vi "Lab Panel V6.00.vi"() -> ()   [LabVIEW 2017] (continued)
                            n1789 = local write "mail control"("END") -> ()
                            n1790 = Bundle(cluster=w3343) -> (w3344:T4)  [unwired: 3 in]
                            n1791 = local write "RUN LAB05-2"(w3341) -> ()
                            n1792 = local write "O/I  LAB05-2"(w3341) -> ()
                            n1793 = local write "run lab05-2"(w3341) -> ()
                            n1794 = local write "DISP LAB05-2"(w3344) -> ()
                          }
                          frame #1 {
                            n1795 = TDMS Close(11:w3345) -> (0:w3346:errorcluster)  [unwired: 1 in, 1 out]
                            n1796 = local write "data file error"(w3346) -> ()
                          }
                          frame #2 {
                            n1797 = stacked-sequence {
                              tunnel: "LAB05-2" -> [w3354 w3360]
                              tunnel: w3351 -> [_ w3359]
                              tunnel: w3350 -> [_ w3358]
                              tunnel: w3349 -> [_ w3357]
                              tunnel: w3348 -> [_ w3356]
                              tunnel: w3347 -> [_ w3355]
                              frame #0 {
                                n1798 = call "sub vi - defrag tdms v1.vi"("panel id"=w3354) -> ("error out"=w3353:errorcluster)  [unwired: 10 in]
                                n1799 = local write "data file error"(w3353) -> ()
                              }
                              frame #1 {
                                n1800 = Bundle("STATUS"=w3359, "OUT SERVER ADDRESS"=w3358, "FROM ACCOUNT"=w3357, "Mail Test File To:"=w3356, "Mail Test Fail"=w3355) -> (w3362:T29)  [unwired: 1 in]
                                n1801 = call "Save data file (pass-fail) v5.vi"("Input Cluster"=w3362, "panel id"=w3360) -> ("network file save error"=w3361:errorcluster)  [unwired: 8 in, 1 out]
                                n1802 = local write "data file error"(w3361) -> ()
                              }
                            }
                          }
                        }
                      }
                    }
                  }
                }
              }
            }
            n1803 = global write "Global display 2.vi" "Mail test file to:"(w2869) -> ()
            n1804 = local read "Network Directory"() -> (w2875:path)
            n1805 = global write "Global 1.vi" "Network Drive"(w2875) -> ()
          }
          frame #8 {
            # "disable functions"
            n1806 = stacked-sequence {
              tunnel: w3372 -> [w3386 _ w3443]
              tunnel: w3371 -> [w3381 _ w3442]
              tunnel: w3370 -> [w3380 _ w3441]
              tunnel: w3369 -> [w3378 _ w3440]
              tunnel: w3368 -> [w3379 _ w3439]
              tunnel: w3367 -> [_ w3403 w3438]
              tunnel: w3366 -> [_ w3404 w3437]
              tunnel: w3365 -> [_ w3405 w3436]
              tunnel: w3364 -> [_ w3406 w3435]
              tunnel: w3363 -> [_ w3407 w3434]
              frame #0 {
                n1807 = Select(t=2, s=w3378, f=0) -> (s? t:f=w3374:i32)
                n1808 = Select(t=2, s=w3380, f=0) -> (s? t:f=w3375:i32)
                n1809 = Select(t=2, s=w3379, f=0) -> (s? t:f=w3373:i32)
                n1810 = Select(t=2, s=w3386, f=0) -> (s? t:f=w3377:i32)
                n1811 = Select(t=2, s=w3381, f=0) -> (s? t:f=w3376:i32)
                n1812 = property on="SELECT LAB02-2" class="RadioBtnsControl (strict)"("DisabledEnum"=w3374) -> ()  [unwired: 2 in, 2 out]
                n1813 = property on="SELECT LAB02-1" class="RadioBtnsControl (strict)"("DisabledEnum"=w3375) -> ()  [unwired: 2 in, 2 out]
                n1814 = property on="SELECT LAB03-1" class="RadioBtnsControl (strict)"("DisabledEnum"=w3373) -> ()  [unwired: 2 in, 2 out]
                n1815 = property on="SELECT LAB01-1" class="RadioBtnsControl (strict)"("DisabledEnum"=w3377) -> ()  [unwired: 2 in, 2 out]
                n1816 = property on="SELECT LAB01-2" class="RadioBtnsControl (strict)"("DisabledEnum"=w3376) -> ()  [unwired: 2 in, 2 out]
                n1817 = Not(x=w3386) -> (.not. x?=w3387:bool)
                n1818 = property on="RESULT LAB01-1" class="Bool (strict)"("Visible"=w3387) -> ()  [unwired: 2 in, 2 out]
                n1819 = Not(x=w3381) -> (.not. x?=w3385:bool)
                n1820 = Not(x=w3380) -> (.not. x?=w3384:bool)
                n1821 = Not(x=w3378) -> (.not. x?=w3383:bool)
                n1822 = property on="RESULT LAB01-2" class="Bool (strict)"("Visible"=w3385) -> ()  [unwired: 2 in, 2 out]
                n1823 = Not(x=w3379) -> (.not. x?=w3382:bool)
                n1824 = property on="RESULT LAB02-1" class="Bool (strict)"("Visible"=w3384) -> ()  [unwired: 2 in, 2 out]
                n1825 = property on="RESULT LAB02-2" class="Bool (strict)"("Visible"=w3383) -> ()  [unwired: 2 in, 2 out]
                n1826 = property on="RESULT LAB03-1" class="Bool (strict)"("Visible"=w3382) -> ()  [unwired: 2 in, 2 out]
                n1827 = property on="SET LAB01-1" class="Clust (strict)"("DisabledEnum"=w3377) -> ()  [unwired: 2 in, 2 out]
                n1828 = property on="SET LAB01-2" class="Clust (strict)"("DisabledEnum"=w3376) -> ()  [unwired: 2 in, 2 out]
                n1829 = property on="SET LAB02-1" class="Clust (strict)"("DisabledEnum"=w3375) -> ()  [unwired: 2 in, 2 out]
                n1830 = property on="SET LAB02-2" class="Clust (strict)"("DisabledEnum"=w3374) -> ()  [unwired: 2 in, 2 out]
                n1831 = property on="SET LAB03-1" class="Clust (strict)"("DisabledEnum"=w3373) -> ()  [unwired: 2 in, 2 out]
                n1832 = property on="O/I  LAB01-1" class="Bool (strict)"("DisabledEnum"=w3377) -> ()  [unwired: 2 in, 2 out]
                n1833 = property on="O/I  LAB01-2" class="Bool (strict)"("DisabledEnum"=w3376) -> ()  [unwired: 2 in, 2 out]
                n1834 = property on="O/I  LAB02-1" class="Bool (strict)"("DisabledEnum"=w3375) -> ()  [unwired: 2 in, 2 out]
                n1835 = property on="O/I  LAB02-2" class="Bool (strict)"("DisabledEnum"=w3374) -> ()  [unwired: 2 in, 2 out]
                n1836 = property on="O/I  LAB03-1" class="Bool (strict)"("DisabledEnum"=w3373) -> ()  [unwired: 2 in, 2 out]
              }
              frame #1 {
                n1837 = Select(t=2, s=w3407, f=0) -> (s? t:f=w3398:i32)
                n1838 = Select(t=2, s=w3406, f=0) -> (s? t:f=w3399:i32)
                n1839 = Select(t=2, s=w3403, f=0) -> (s? t:f=w3402:i32)
                n1840 = Select(t=2, s=w3404, f=0) -> (s? t:f=w3401:i32)
                n1841 = Select(t=2, s=w3405, f=0) -> (s? t:f=w3400:i32)
                n1842 = property on="SELECT LAB05-2" class="RadioBtnsControl (strict)"("DisabledEnum"=w3398) -> ()  [unwired: 2 in, 2 out]
                n1843 = property on="SELECT LAB05-1" class="RadioBtnsControl (strict)"("DisabledEnum"=w3399) -> ()  [unwired: 2 in, 2 out]
                n1844 = property on="SELECT LAB03-2" class="RadioBtnsControl (strict)"("DisabledEnum"=w3402) -> ()  [unwired: 2 in, 2 out]
                n1845 = property on="SELECT LAB04-1" class="RadioBtnsControl (strict)"("DisabledEnum"=w3401) -> ()  [unwired: 2 in, 2 out]
                n1846 = property on="SELECT LAB04-2" class="RadioBtnsControl (strict)"("DisabledEnum"=w3400) -> ()  [unwired: 2 in, 2 out]
                n1847 = property on="SET LAB05-2" class="Clust (strict)"("DisabledEnum"=w3398) -> ()  [unwired: 2 in, 2 out]
                n1848 = property on="SET LAB05-1" class="Clust (strict)"("DisabledEnum"=w3399) -> ()  [unwired: 2 in, 2 out]
                n1849 = property on="SET LAB03-2" class="Clust (strict)"("DisabledEnum"=w3402) -> ()  [unwired: 2 in, 2 out]
                n1850 = property on="SET LAB04-1" class="Clust (strict)"("DisabledEnum"=w3401) -> ()  [unwired: 2 in, 2 out]
                n1851 = property on="SET LAB04-2" class="Clust (strict)"("DisabledEnum"=w3400) -> ()  [unwired: 2 in, 2 out]
                n1852 = property on="O/I  LAB05-2" class="Bool (strict)"("DisabledEnum"=w3398) -> ()  [unwired: 2 in, 2 out]
                n1853 = property on="O/I  LAB05-1" class="Bool (strict)"("DisabledEnum"=w3399) -> ()  [unwired: 2 in, 2 out]
                n1854 = property on="O/I  LAB04-1" class="Bool (strict)"("DisabledEnum"=w3401) -> ()  [unwired: 2 in, 2 out]
                n1855 = property on="O/I  LAB04-2" class="Bool (strict)"("DisabledEnum"=w3400) -> ()  [unwired: 2 in, 2 out]
                n1856 = property on="O/I  LAB03-2" class="Bool (strict)"("DisabledEnum"=w3402) -> ()  [unwired: 2 in, 2 out]
                n1857 = Not(x=w3407) -> (.not. x?=w3408:bool)
                n1858 = Not(x=w3406) -> (.not. x?=w3409:bool)
                n1859 = Not(x=w3405) -> (.not. x?=w3410:bool)
                n1860 = property on="RESULT LAB05-2" class="Bool (strict)"("Visible"=w3408) -> ()  [unwired: 2 in, 2 out]
                n1861 = property on="RESULT LAB05-1" class="Bool (strict)"("Visible"=w3409) -> ()  [unwired: 2 in, 2 out]
                n1862 = Not(x=w3404) -> (.not. x?=w3411:bool)
                n1863 = property on="RESULT LAB04-2" class="Bool (strict)"("Visible"=w3410) -> ()  [unwired: 2 in, 2 out]
                n1864 = Not(x=w3403) -> (.not. x?=w3412:bool)
                n1865 = property on="RESULT LAB04-1" class="Bool (strict)"("Visible"=w3411) -> ()  [unwired: 2 in, 2 out]
                n1866 = property on="RESULT LAB03-2" class="Bool (strict)"("Visible"=w3412) -> ()  [unwired: 2 in, 2 out]
              }
              frame #2 {
                # "disable calibrate if any test running"
                n1867 = Or(x=w3435, y=w3434) -> (x .or. y?=w3428:bool)
                n1868 = Or(x=w3437, y=w3436) -> (x .or. y?=w3430:bool)
                n1869 = Or(x=w3441, y=w3440) -> (x .or. y?=w3432:bool)
                n1870 = Or(x=w3439, y=w3438) -> (x .or. y?=w3431:bool)
                n1871 = Or(x=w3443, y=w3442) -> (x .or. y?=w3433:bool)
                n1872 = Or(x=w3431, y=w3430) -> (x .or. y?=w3429:bool)
                n1873 = Or(x=w3433, y=w3432) -> (x .or. y?=w3427:bool)
                n1874 = Or(x=w3429, y=w3428) -> (x .or. y?=w3426:bool)
                n1875 = Or(x=w3427, y=w3426) -> (x .or. y?=w3423:bool)
                "Any Test Running" <- w3423
                n1876 = case shown="False" w3423 {
                  tunnel: [0 2] -> w3425
                  frame False {
                  }
                  frame True {
                  }
                }
                n1877 = property on="JIG TEST" class="Clust (strict)"("DisabledEnum"=w3425) -> ()  [unwired: 2 in, 2 out]
                n1878 = property on="Network Directory" class="Path"("DisabledEnum"=w3425) -> ()  [unwired: 2 in, 2 out]
                n1879 = property on="MAIL SETTINGS" class="Clust (strict)"("DisabledEnum"=w3425) -> ()  [unwired: 2 in, 2 out]
                n1880 = property on="SET (cal)" class="Bool (strict)"("DisabledEnum"=w3425) -> ()  [unwired: 2 in, 2 out]
                n1881 = property on="ADMIN" class="Bool (strict)"("DisabledEnum"=0) -> ()  [unwired: 2 in, 2 out]
              }
            }
          }
          frame #9 {
            # "Note : JIG LAB0X-N   are written to digital I/O in frame 11"
            # "Drive jigs"
            n1882 = stacked-sequence {
              frame #0 {
                # "jig on"
                n1883 = local read "jig cycle"() -> (w3451:dbl)
                n1884 = property on="JIG TEST" class="Clust (strict)"() -> ("DisabledEnum"=w3448:T17)  [unwired: 2 in, 2 out]
                n1885 = Equal?(x=w3448, y=2) -> (x = y?=w3447:bool)
                n1886 = Equal?(x=w3451, y=0) -> (x = y?=w3449:bool)
                n1887 = And(x=w3449, y=w3447) -> (x .and. y?=w3446:bool)
                n1888 = case shown="True" w3446 {
                  frame False {
                  }
                  frame True {
                    n1889 = local read "run lab01-2"() -> (w3461:bool)
                    n1890 = local read "run lab01-1"() -> (w3462:bool)
                    n1891 = local read "run lab02-1"() -> (w3460:bool)
                    n1892 = local read "run lab02-2"() -> (w3459:bool)
                    n1893 = local read "run lab03-1"() -> (w3458:bool)
                    n1894 = local read "run lab03-2"() -> (w3457:bool)
                    n1895 = local read "run lab04-1"() -> (w3456:bool)
                    n1896 = local read "run lab04-2"() -> (w3455:bool)
                    n1897 = local read "run lab05-1"() -> (w3454:bool)
                    n1898 = local read "run lab05-2"() -> (w3453:bool)
                    n1899 = local write "JIG LAB01-2"(w3461) -> ()
                    n1900 = local write "JIG LAB03-2"(w3457) -> ()
                    n1901 = local write "JIG LAB01-1"(w3462) -> ()
                    n1902 = local write "JIG LAB02-1"(w3460) -> ()
                    n1903 = local write "JIG LAB02-2"(w3459) -> ()
                    n1904 = local write "JIG LAB03-1"(w3458) -> ()
                    n1905 = local write "JIG LAB04-1"(w3456) -> ()
                    n1906 = local write "JIG LAB04-2"(w3455) -> ()
                    n1907 = local write "JIG LAB05-1"(w3454) -> ()
                    n1908 = local write "JIG LAB05-2"(w3453) -> ()
                  }
                }
              }
              frame #1 {
                # "jig off"
                n1909 = local read "jig cycle"() -> (w3469:dbl)
                n1910 = local read "on loops"() -> (w3468:dbl)
                n1911 = property on="JIG TEST" class="Clust (strict)"() -> ("DisabledEnum"=w3467:T17)  [unwired: 2 in, 2 out]
                n1912 = Equal?(x=w3467, y=2) -> (x = y?=w3465:bool)
                n1913 = Equal?(x=w3469, y=w3468) -> (x = y?=w3464:bool)
                n1914 = And(x=w3464, y=w3465) -> (x .and. y?=w3463:bool)
                n1915 = case shown="True" w3463 {
                  frame False {
                  }
                  frame True {
                    w3520 = FALSE
                    w3521 = TRUE
                    w3519 = 2
                    n1916 = local read "SELECT LAB05-2"() -> (w3510:T3)
                    n1917 = local read "SELECT LAB04-2"() -> (w3512:T3)
                    n1918 = local read "SELECT LAB04-1"() -> (w3513:T3)
                    n1919 = local read "SELECT LAB05-1"() -> (w3511:T3)
                    n1920 = local read "SELECT LAB03-2"() -> (w3514:T3)
                    n1921 = local read "SELECT LAB02-1"() -> (w3517:T3)
                    n1922 = local read "SELECT LAB03-1"() -> (w3515:T3)
                    n1923 = local read "SELECT LAB02-2"() -> (w3516:T3)
                    n1924 = local read "SELECT LAB01-2"() -> (w3518:T3)
                    n1925 = local read "run lab05-1"() -> (w3480:bool)
                    n1926 = local read "run lab05-2"() -> (w3479:bool)
                    n1927 = local read "run lab04-2"() -> (w3481:bool)
                    n1928 = local read "SELECT LAB01-1"() -> (w3522:T3)
                    n1929 = local read "run lab04-1"() -> (w3482:bool)
                    n1930 = local read "run lab01-1"() -> (w3498:bool)
                    n1931 = local read "run lab01-2"() -> (w3487:bool)
                    n1932 = local read "run lab03-2"() -> (w3483:bool)
                    n1933 = local read "run lab03-1"() -> (w3484:bool)
                    n1934 = local read "run lab02-1"() -> (w3486:bool)
                    n1935 = local read "run lab02-2"() -> (w3485:bool)
                    n1936 = Equal?(x=w3519, y=w3515) -> (x = y?=w3493:bool)
                    n1937 = Equal?(x=w3519, y=w3514) -> (x = y?=w3492:bool)
                    n1938 = Equal?(x=w3519, y=w3513) -> (x = y?=w3491:bool)
                    n1939 = Equal?(x=w3519, y=w3512) -> (x = y?=w3490:bool)
                    n1940 = Equal?(x=w3519, y=w3511) -> (x = y?=w3489:bool)
                    n1941 = Equal?(x=w3519, y=w3510) -> (x = y?=w3488:bool)
                    n1942 = Equal?(x=w3519, y=w3522) -> (x = y?=w3499:bool)
                    n1943 = Equal?(x=w3519, y=w3517) -> (x = y?=w3495:bool)
                    n1944 = Equal?(x=w3519, y=w3516) -> (x = y?=w3494:bool)
                    n1945 = Equal?(x=w3519, y=w3518) -> (x = y?=w3496:bool)
                    n1946 = And(x=w3490, y=w3481) -> (x .and. y?=w3472:bool)
                    n1947 = And(x=w3493, y=w3484) -> (x .and. y?=w3475:bool)
                    n1948 = And(x=w3491, y=w3482) -> (x .and. y?=w3473:bool)
                    n1949 = And(x=w3488, y=w3479) -> (x .and. y?=w3470:bool)
                    n1950 = And(x=w3494, y=w3485) -> (x .and. y?=w3476:bool)
                    n1951 = And(x=w3492, y=w3483) -> (x .and. y?=w3474:bool)
                    n1952 = And(x=w3489, y=w3480) -> (x .and. y?=w3471:bool)
                    n1953 = And(x=w3496, y=w3487) -> (x .and. y?=w3478:bool)
                    n1954 = And(x=w3499, y=w3498) -> (x .and. y?=w3497:bool)
                    n1955 = And(x=w3495, y=w3486) -> (x .and. y?=w3477:bool)
                    n1956 = Select(t=w3521, s=w3497, f=w3520) -> (s? t:f=w3500:bool)
                    n1957 = Select(t=w3521, s=w3478, f=w3520) -> (s? t:f=w3501:bool)
                    n1958 = Select(t=w3521, s=w3477, f=w3520) -> (s? t:f=w3502:bool)
                    n1959 = Select(t=w3521, s=w3476, f=w3520) -> (s? t:f=w3503:bool)
                    n1960 = Select(t=w3521, s=w3475, f=w3520) -> (s? t:f=w3504:bool)
                    n1961 = Select(t=w3521, s=w3474, f=w3520) -> (s? t:f=w3505:bool)
                    n1962 = Select(t=w3521, s=w3473, f=w3520) -> (s? t:f=w3506:bool)
                    n1963 = Select(t=w3521, s=w3472, f=w3520) -> (s? t:f=w3507:bool)
                    n1964 = Select(t=w3521, s=w3471, f=w3520) -> (s? t:f=w3508:bool)
                    n1965 = Select(t=w3521, s=w3470, f=w3520) -> (s? t:f=w3509:bool)
                    n1966 = local write "JIG LAB03-2"(w3505) -> ()
                    n1967 = local write "JIG LAB02-1"(w3502) -> ()
                    n1968 = local write "JIG LAB02-2"(w3503) -> ()
                    n1969 = local write "JIG LAB01-2"(w3501) -> ()
                    n1970 = local write "JIG LAB03-1"(w3504) -> ()
                    n1971 = local write "JIG LAB01-1"(w3500) -> ()
                    n1972 = local write "JIG LAB05-2"(w3509) -> ()
                    n1973 = local write "JIG LAB04-1"(w3506) -> ()
                    n1974 = local write "JIG LAB05-1"(w3508) -> ()
                    n1975 = local write "JIG LAB04-2"(w3507) -> ()
                  }
                }
              }
            }
          }
          frame #10 {
            # "Note : JIG LAB0X-N   are written to digital I/O in frame 11"
            # "enable  jig test output if no test busy"
            n1976 = property on="JIG TEST" class="Clust (strict)"() -> ("DisabledEnum"=w3525:T17)  [unwired: 2 in, 2 out]
            n1977 = Equal?(x=w3525, y=0) -> (x = y?=w3523:bool)
            n1978 = case shown="True" w3523 {
              frame False {
              }
              frame True {
                n1979 = local read "JIG TEST"() -> (w3536:T11)
                n1980 = Unbundle(w3536) -> ("LAB01-1"=w3535:bool, "LAB01-2"=w3534:bool, "LAB02-1"=w3533:bool, "LAB02-2"=w3532:bool, "LAB03-1"=w3531:bool, "LAB03-2"=w3530:bool, "LAB04-1"=w3529:bool, "LAB04-2"=w3528:bool, "LAB05-1"=w3527:bool, "LAB05-2"=w3526:bool)
                n1981 = local write "JIG LAB05-1"(w3527) -> ()
                n1982 = local write "JIG LAB05-2"(w3526) -> ()
                n1983 = local write "JIG LAB04-1"(w3529) -> ()
                n1984 = local write "JIG LAB04-2"(w3528) -> ()
                n1985 = local write "JIG LAB03-2"(w3530) -> ()
                n1986 = local write "JIG LAB01-1"(w3535) -> ()
                n1987 = local write "JIG LAB02-1"(w3533) -> ()
                n1988 = local write "JIG LAB03-1"(w3531) -> ()
                n1989 = local write "JIG LAB01-2"(w3534) -> ()
                n1990 = local write "JIG LAB02-2"(w3532) -> ()
              }
            }
          }
          frame #11 {
            w3537 = FALSE
            # "Drive digital output and reset USB and temperature network if required."
            n1991 = global read "Global display 3.vi" "cycle O/F"() -> (w3546:bool)
            n1992 = case shown="False" w3546 {
              tunnel: [w3678 FALSE] -> w3545
              frame False {
                n1993 = local read "Analog error"() -> (w3680:bool)
                n1994 = local read "Reset Measuring"() -> (w3679:bool)
                n1995 = Or(x=w3679, y=w3680) -> (x .or. y?=w3678:bool)
              }
              frame True {
              }
            }
            n1996 = local read "O/I  LAB01-1"() -> (w3565:bool)
            n1997 = local read "JIG LAB01-1"() -> (w3564:bool)
            n1998 = local read "O/I  LAB01-2"() -> (w3563:bool)
            n1999 = local read "JIG LAB01-2"() -> (w3562:bool)
            n2000 = local read "O/I  LAB02-1"() -> (w3561:bool)
            n2001 = local read "JIG LAB02-1"() -> (w3560:bool)
            n2002 = local read "O/I  LAB02-2"() -> (w3559:bool)
            n2003 = local read "JIG LAB02-2"() -> (w3558:bool)
            n2004 = local read "O/I  LAB03-1"() -> (w3557:bool)
            n2005 = local read "JIG LAB03-1"() -> (w3556:bool)
            n2006 = local read "O/I  LAB03-2"() -> (w3555:bool)
            n2007 = local read "JIG LAB03-2"() -> (w3554:bool)
            n2008 = local read "O/I  LAB04-1"() -> (w3553:bool)
            n2009 = local read "JIG LAB04-1"() -> (w3552:bool)
            n2010 = local read "O/I  LAB04-2"() -> (w3543:bool)
            n2011 = local read "JIG LAB04-2"() -> (w3542:bool)
            n2012 = local read "O/I  LAB05-1"() -> (w3541:bool)
            n2013 = local read "JIG LAB05-1"() -> (w3540:bool)
            n2014 = local read "O/I  LAB05-2"() -> (w3539:bool)
            n2015 = local read "JIG LAB05-2"() -> (w3538:bool)
            n2016 = Build Array(w3558, w3557, w3556, w3555, w3554, w3553, w3552) -> (w3550:bool[])
            "USB OUT 1" <- w3550
            n2017 = Build Array(w3565, w3564, w3563, w3562, w3561, w3560, w3559) -> (w3551:bool[])
            "USB OUT 0" <- w3551
            n2018 = Build Array(w3543, w3542, w3541, w3540, w3539, w3538, w3537, w3537) -> (w3549:bool[])
            "USB OUT 2" <- w3549
            n2019 = Not(x=w3546) -> (.not. x?=w3547:bool)
            n2020 = local read "Simulate"() -> (w3548:bool)
            n2021 = And(x=w3547, y=w3545) -> (x .and. y?=w3544:bool)
            n2022 = stacked-sequence {
              tunnel: w3551 -> [w3569 w3575]
              tunnel: w3550 -> [w3568 w3574]
              tunnel: w3549 -> [w3567 w3573]
              tunnel: w3548 -> [w3566 w3576]
              tunnel: w3544 -> [_ w3577]
              frame #0 {
                # "drive outputs for normal use"
                n2023 = case shown="False" w3566 {
                  tunnel: w3569 -> [w3572 _]
                  tunnel: w3568 -> [w3571 _]
                  tunnel: w3567 -> [w3570 _]
                  frame False {
                    n2024 = call "sub vi - Drive Relays All v6.vi"("Array #2"=w3570, "Array #1"=w3571, "Array #0"=w3572) -> ()  [unwired: 8 in, 1 out]
                  }
                  frame True {
                  }
                }
              }
              frame #1 {
                # "USB  reset routine"
                n2025 = case shown="True" w3577 {
                  tunnel: w3576 -> [_ w3581]
                  tunnel: w3575 -> [_ w3580]
                  tunnel: w3574 -> [_ w3579]
                  tunnel: w3573 -> [_ w3578]
                  frame False {
                  }
                  frame True {
                    n2026 = stacked-sequence {
                      seq-local: [w3583 _ _ _ _] -> [_ w3589 _ _ _]
                      tunnel: w3581 -> [_ w3593 _ _ _]
                      tunnel: w3580 -> [_ w3592 _ _ _]
                      tunnel: w3579 -> [_ w3591 _ _ _]
                      tunnel: w3578 -> [_ w3590 _ _ _]
                      frame #0 {
                        n2027 = case shown="False" "Auto Reset" {
                          tunnel: [w3586 FALSE] -> w3584
                          frame False {
                            n2028 = Two Button Dialog(message="System reset") -> (T button?=w3586:bool)  [unwired: 2 in]
                          }
                          frame True {
                          }
                        }
                        n2029 = disable-structure shown="Disabled" {
                          frame Disabled {
                            n2030 = local write "Tab Control 2"(5) -> ()
                          }
                          frame Enabled {
                          }
                        }
                        n2031 = Or(x="Auto Reset", y=w3584) -> (x .or. y?=w3583:bool)
                      }
                      frame #1 {
                        n2032 = case shown="True" w3589 {
                          tunnel: w3593 -> [_ w3599]
                          tunnel: w3592 -> [_ w3598]
                          tunnel: w3591 -> [_ w3597]
                          tunnel: w3590 -> [_ w3596]
                          frame False {
                          }
                          frame True {
                            n2033 = stacked-sequence {
                              tunnel: w3599 -> [_ w3617 _]
                              tunnel: bool[] [] -> [w3602 w3616 w3635]
                              tunnel: w3598 -> [_ _ w3634]
                              tunnel: w3597 -> [w3601 _ w3633]
                              tunnel: w3596 -> [w3600 _ w3632]
                              tunnel: 5000 -> [w3603 _ w3631]
                              frame #0 {
                                # "switch off test stations for system reset"
                                n2034 = stacked-sequence {
                                tunnel: w3603 -> [w3607 w3611 w3613]
                                tunnel: w3602 -> [w3606 w3610 w3614]
                                tunnel: w3601 -> [w3605 _ _]
                                tunnel: w3600 -> [w3604 w3609 _]
                                frame #0 {
                                # "drive 1st 7 inputs"
                                n2035 = call "sub vi - Drive Relays All v6.vi"("Array #2"=w3604, "Array #1"=w3605, "Array #0"=w3606) -> ()  [unwired: 8 in, 1 out]
                                n2036 = call "Message Display V1.vi"("Message"="Delay off LAB 01-1 to 02-1", "Delay mS"=w3607) -> ()  [unwired: 10 in]
                                }
                                frame #1 {
                                # "drive 2nd 7 inputs"
                                n2037 = call "sub vi - Drive Relays All v6.vi"("Array #2"=w3609, "Array #1"=w3610, "Array #0"=w3610) -> ()  [unwired: 8 in, 1 out]
                                n2038 = call "Message Display V1.vi"("Message"="Delay off LAB 02-2 to 04-1", "Delay mS"=w3611) -> ()  [unwired: 10 in]
                                }
                                frame #2 {
                                # "drive 3rd 7 inputs"
                                n2039 = call "sub vi - Drive Relays All v6.vi"("Array #2"=w3614, "Array #1"=w3614, "Array #0"=w3614) -> ()  [unwired: 8 in, 1 out]
                                n2040 = call "Message Display V1.vi"("Message"="Delay off LAB 04-2 to 05-2", "Delay mS"=w3613) -> ()  [unwired: 10 in]
                                }
                                }
                              }
                              frame #1 {
                                # "reset all usb modules"
                                n2041 = stacked-sequence {
                                tunnel: w3617 -> [_ w3622]
                                tunnel: w3616 -> [w3620 _]
                                frame #0 {
                                n2042 = local write "AI Task"(FALSE) -> ()
                                n2043 = call "sub vi - Drive Relays All v6.vi"("Array #2"=bool[] [FALSE, FALSE, FALSE, FALSE, FALSE, FALSE, TRUE, FALSE], "Array #1"=w3620, "Array #0"=w3620) -> ()  [unwired: 8 in, 1 out]
                                }
                                frame #1 {
                                n2044 = call "Reset Meas v 5.vi"("simulate"=w3622) -> ("Reset Error"=w3621:bool)  [unwired: 10 in]
                                n2045 = case shown="False" w3621 {
                                frame False {
                                n2046 = local read "RATE (Hz)"() -> (w3626:dbl)
                                n2047 = local read "SAMPLES"() -> (w3625:dbl)
                                n2048 = call "sub vi - AI USB4704 (3)  Create Task v4.vi"("Rate Hz"=w3626, "Samples"=w3625) -> ("TASK USB 0"=w3629:i32, "TASK USB 1"=w3628:i32, "TASK USB 2"=w3627:i32, "AI Task Er"=w3623:bool)  [unwired: 9 in, 1 out]
                                n2049 = local write "AI Task"(TRUE) -> ()
                                n2050 = local write "Reset Error"(w3623) -> ()
                                n2051 = local write "AI Task2"(w3627) -> ()
                                n2052 = local write "AI Task1"(w3628) -> ()
                                n2053 = local write "AI Task0"(w3629) -> ()
                                }
                                frame True {
                                "Reset Error" <- TRUE
                                }
                                }
                                }
                                }
                              }
                              frame #2 {
                                # "switch test stations back on after reset"
                                n2054 = stacked-sequence {
                                tunnel: w3635 -> [w3639 w3642 _]
                                tunnel: w3634 -> [w3638 w3644 w3649]
                                tunnel: w3631 -> [w3637 w3640 w3646]
                                tunnel: w3633 -> [_ w3643 w3648]
                                tunnel: w3632 -> [_ _ w3645]
                                frame #0 {
                                # "drive 1st 7 inputs"
                                n2055 = call "sub vi - Drive Relays All v6.vi"("Array #2"=w3639, "Array #1"=w3639, "Array #0"=w3638) -> ()  [unwired: 8 in, 1 out]
                                n2056 = call "Message Display V1.vi"("Message"="Delay on LAB 01-1 to 02-1", "Delay mS"=w3637) -> ()  [unwired: 10 in]
                                }
                                frame #1 {
                                # "drive 1st & 2nd outputs"
                                n2057 = call "sub vi - Drive Relays All v6.vi"("Array #2"=w3642, "Array #1"=w3643, "Array #0"=w3644) -> ()  [unwired: 8 in, 1 out]
                                n2058 = call "Message Display V1.vi"("Message"="Delay on LAB 02-2 to 04-1", "Delay mS"=w3640) -> ()  [unwired: 10 in]
                                }
                                frame #2 {
                                n2059 = call "sub vi - Drive Relays All v6.vi"("Array #2"=w3645, "Array #1"=w3648, "Array #0"=w3649) -> ()  [unwired: 8 in, 1 out]
                                n2060 = call "Message Display V1.vi"("Message"="Delay on LAB 04-2 to 05-2", "Delay mS"=w3646) -> ()  [unwired: 10 in]
                                }
                                }
                              }
                            }
                          }
                        }
                      }
                      frame #2 {
                        w3650 = 0
                        w3651 = FALSE
                        # "set all back to zero"
                        n2061 = local read "Total USB resets"() -> (w3653:dbl)
                        n2062 = local read "Resets Done"() -> (w3655:dbl)
                        n2063 = local write "Reset Measuring"(w3651) -> ()
                        n2064 = local write "Analog error"(w3651) -> ()
                        n2065 = local write "Er USB#2"(w3650) -> ()
                        n2066 = local write "Er USB#0"(w3650) -> ()
                        n2067 = local write "Er USB#1"(w3650) -> ()
                        n2068 = local write "Error USB #0"(w3651) -> ()
                        n2069 = local write "Error USB #1"(w3651) -> ()
                        n2070 = local write "Error USB #2"(w3651) -> ()
                        n2071 = Increment(x=w3653) -> (x+1=w3652:dbl)
                        n2072 = Increment(x=w3655) -> (x+1=→"Resets Done":dbl)
                        n2073 = local write "Total USB resets"(w3652) -> ()
                      }
                      frame #3 {
                        # "save reset value"
                        n2074 = String To Path(string="c:\\crabtree\\Set Up\\") -> (path=w3665:path)
                        n2075 = Build Path(base path=w3665, name or relative path="USB resets.bin") -> (appended path=w3658:path)
                        n2076 = Create Folder(path (use dialog)=w3665) -> (error out=w3657:errorcluster)  [unwired: 2 in, 2 out]
                        n2077 = local read "Total USB resets"() -> (w3656:dbl)
                        n2078 = call <vilib>:"Clear Errors.vi"("error in (no error)"=w3657) -> ()  [unwired: 5 in, 2 out]
                        n2079 = Open/Create/Replace File(file path (use dialog)=w3658, operation (0:open)=T18."replace or create") -> (refnum out=w3663:refnum<file>, error out=w3662:errorcluster)  [unwired: 4 in, 1 out]
                        n2080 = Write to Binary File(file (use dialog)=w3663, data=w3656, error in=w3662) -> (refnum out=w3661:refnum<file>, error out=w3660:errorcluster)  [unwired: 3 in, 1 out]
                        n2081 = Close File(refnum=w3661, error in=w3660) -> (error out=w3659:errorcluster)  [unwired: 1 out]
                        n2082 = local write "data file error"(w3659) -> ()
                      }
                      frame #4 {
                        # "mail reset value"
                        n2083 = local read "MAIL SETTINGS"() -> (w3671:T8)
                        n2084 = local read "Total USB resets"() -> (w3675:dbl)
                        n2085 = Unbundle(w3671) -> ("OUT SERVER ADDRESS"=w3677:string, "FROM ACCOUNT"=w3676:string)  [unwired: 5 out]
                        n2086 = Number To Decimal String(number=w3675) -> (decimal integer string=w3673:string)  [unwired: 1 in]
                        n2087 = Concatenate Strings("Total USB resets: ", w3673) -> (w3672:string)
                        n2088 = call "sub vi - send mail v5.vi"("TO:"="francois@ffg.net", "subject"=w3672, "from"=w3676, "out going server"=w3677) -> ("error out"=w3670:errorcluster)  [unwired: 11 in]
                        n2089 = Bundle(cluster=w3671, "mail error"=w3670) -> (w3669:T8)  [unwired: 6 in]
                        n2090 = local write "MAIL SETTINGS"(w3669) -> ()
                      }
                    }
                  }
                }
              }
            }
          }
          frame #12 {
            # "if all test panels are off stop analog read"
            n2091 = local read "O/I  LAB03-1"() -> (w3703:bool)
            n2092 = local read "O/I  LAB03-2"() -> (w3702:bool)
            n2093 = local read "O/I  LAB04-1"() -> (w3701:bool)
            n2094 = local read "O/I  LAB04-2"() -> (w3700:bool)
            n2095 = local read "O/I  LAB05-1"() -> (w3699:bool)
            n2096 = local read "O/I  LAB05-2"() -> (w3698:bool)
            n2097 = local read "O/I  LAB02-2"() -> (w3704:bool)
            n2098 = local read "O/I  LAB02-1"() -> (w3705:bool)
            n2099 = local read "O/I  LAB01-2"() -> (w3706:bool)
            n2100 = local read "O/I  LAB01-1"() -> (w3707:bool)
            n2101 = Or(x=w3699, y=w3698) -> (x .or. y?=w3696:bool)
            n2102 = Or(x=w3701, y=w3700) -> (x .or. y?=w3697:bool)
            n2103 = Or(x=w3705, y=w3704) -> (x .or. y?=w3695:bool)
            n2104 = Or(x=w3703, y=w3702) -> (x .or. y?=w3693:bool)
            n2105 = Or(x=w3707, y=w3706) -> (x .or. y?=w3694:bool)
            n2106 = Or(x=w3697, y=w3696) -> (x .or. y?=w3690:bool)
            n2107 = Or(x=w3694, y=w3695) -> (x .or. y?=w3692:bool)
            n2108 = Or(x=w3692, y=w3693) -> (x .or. y?=w3691:bool)
            n2109 = Or(x=w3691, y=w3690) -> (x .or. y?=w3688:bool)
            n2110 = local read "Any Test Running"() -> (w3689:bool)
            n2111 = local read "AI Task"() -> (w3684:bool)
            n2112 = Or(x=w3688, y=w3689) -> (x .or. y?=w3683:bool)
            n2113 = Not(x=w3683) -> (.not. x?=w3687:bool)
            n2114 = And(x=w3687, y=w3684) -> (x .and. y?=w3686:bool)
            n2115 = Not(x=w3684) -> (.not. x?=w3685:bool)
            n2116 = And(x=w3683, y=w3685) -> (x .and. y?=w3682:bool)
            n2117 = case shown="True" w3686 {
              frame False {
              }
              frame True {
                # "close task if no test"
                n2118 = local write "AI Task"(FALSE) -> ()
                n2119 = call "sub vi - AI USB4704 (3)  Close Task v2.vi"() -> ()  [unwired: 16 in]
              }
            }
            n2120 = case shown="True" w3682 {
              frame False {
              }
              frame True {
                # "create task for test"
                n2121 = local read "SAMPLES"() -> (w3709:dbl)
                n2122 = local read "RATE (Hz)"() -> (w3708:dbl)
                n2123 = call "sub vi - AI USB4704 (3)  Create Task v4.vi"("Rate Hz"=w3708, "Samples"=w3709) -> ("TASK USB 0"=w3710:i32, "TASK USB 1"=w3711:i32, "TASK USB 2"=w3712:i32)  [unwired: 9 in, 2 out]
                n2124 = local write "AI Task0"(w3710) -> ()
                n2125 = local write "AI Task1"(w3711) -> ()
                n2126 = local write "AI Task2"(w3712) -> ()
                n2127 = local write "AI Task"(TRUE) -> ()
              }
            }
          }
          frame #13 {
            # "get all analog values from USB devices"
            n2128 = local read "on loops"() -> (w3722:dbl)
            n2129 = local read "jig cycle"() -> (w3719:dbl)
            n2130 = Add(x=w3722, y=3) -> (x+y=w3720:dbl)
            n2131 = Equal?(x=w3719, y=3) -> (x = y?=w3717:bool)
            n2132 = Equal?(x=w3719, y=w3720) -> (x = y?=w3718:bool)
            n2133 = Or(x=w3717, y=w3718) -> (x .or. y?=w3716:bool)
            n2134 = global write "Global display 3.vi" "cycle O/F"(w3717) -> ()
            n2135 = case shown="True" w3716 {
              tunnel: w3717 -> [_ w3728]
              tunnel: w3715 -> [_ w3725]
              frame False {
              }
              frame True {
                n2136 = local read "Simulate"() -> (w3731:bool)
                n2137 = case shown="False" w3731 {
                  tunnel: [w3747 dynamicdata[] [] ("array GRAPH")] -> w3737
                  tunnel: [w3746 w3772] -> w3736
                  tunnel: [w3745 w3772] -> w3735
                  tunnel: [w3744 w3772] -> w3734
                  tunnel: [w3743 w3772] -> w3733
                  tunnel: [w3742 w3772] -> w3732
                  tunnel: w3728 -> [_ w3776]
                  tunnel: [w3741 "Ambient Volts"] -> w3727
                  tunnel: [w3740 bool[] []] -> w3726
                  tunnel: w3725 -> [w3739 _]
                  tunnel: [w3738 0.3 ("Analog loop time")] -> w3724
                  frame False {
                    # "analog in"
                    n2138 = case shown="True" w3739 {
                      tunnel: [dynamicdata[] [] ("array GRAPH") w3766] -> w3747
                      tunnel: [w3749 w3765] -> w3746
                      tunnel: [w3749 w3764] -> w3745
                      tunnel: [w3749 w3763] -> w3744
                      tunnel: [w3749 w3762] -> w3743
                      tunnel: [w3749 w3761] -> w3742
                      tunnel: [3 w3760] -> w3741
                      tunnel: [bool[] [] w3759] -> w3740
                      tunnel: [0.0 w3755] -> w3738
                      frame False {
                        w3750 = 0.0
                        # "no test"
                        n2139 = Bundle(w3750, w3750, w3750, w3750, w3750, w3750) -> (w3749:cluster{dbl, dbl, dbl, dbl, dbl, dbl})  [unwired: 1 in]
                      }
                      frame True {
                        # "test on"
                        n2140 = local read "AI data 0"() -> (w3758:waveform(dbl)[])
                        n2141 = local read "AI data 1"() -> (w3757:waveform(dbl)[])
                        n2142 = local read "AI data 2"() -> (w3754:waveform(dbl)[])
                        n2143 = local read "AI Error"() -> (w3756:errorcluster[])
                        n2144 = call "sub vi - Read Analog All v9.5.vi"("data 0"=w3758, "data 1"=w3757, "data 2"=w3754, "AI Error"=w3756) -> ("array GRAPH"=w3766:dynamicdata[], "LAB01"=w3765:T30, "LAB02"=w3764:T31, "LAB03"=w3763:T32, "LAB04"=w3762:T33, "deg C"=w3760:dbl, "USB Error"=w3759:bool[], "LAB05"=w3761:T34)  [unwired: 4 in]
                        n2145 = local read "AI loop time"() -> (w3755:dbl)
                      }
                    }
                  }
                  frame True {
                    # "simulate"
                    n2146 = local read "ON amps"() -> (w3770:dbl)
                    n2147 = local read "OFF amps"() -> (w3771:dbl)
                    n2148 = local read "VOLTS"() -> (w3774:dbl)
                    n2149 = local read "PF"() -> (w3773:dbl)
                    n2150 = Select(t=w3770, s=w3776, f=w3771) -> (s? t:f=w3775:dbl)
                    n2151 = Bundle("OFF amps"=w3775, "VOLTS"=w3774, "PF"=w3773, "OFF amps"=w3775, "VOLTS"=w3774, "PF"=w3773) -> (w3772:T35)  [unwired: 1 in]
                  }
                }
                n2152 = local read "Simulate"() -> (w3730:bool)
                n2153 = stacked-sequence {
                  seq-local: [w3780 _ _ _ _ _ _ _] -> [_ _ _ _ _ _ _ _]
                  seq-local: [w3779 _ _ _ _ _ _ _] -> [_ _ _ _ _ _ _ _]
                  seq-local: [w3778 _ _ _ _ _ _ _] -> [_ _ _ _ _ _ _ w3973]
                  tunnel: w3737 -> [_ w3831 _ _ _ _ _ _]
                  tunnel: w3736 -> [_ _ w3858 _ _ _ _ _]
                  tunnel: w3735 -> [_ _ _ w3886 _ _ _ _]
                  tunnel: w3734 -> [_ _ _ _ w3914 _ _ _]
                  tunnel: w3733 -> [_ _ _ _ _ w3942 _ _]
                  tunnel: w3732 -> [_ _ _ _ _ _ w3970 _]
                  tunnel: w3730 -> [_ _ w3857 w3885 w3913 w3941 w3969 w3975]
                  tunnel: T15 {"1  (A) cal"=1.0, "1 (V) cal"=1.0, "1 (PF) cal"=1.0, "1 (TL) cal"=1.0, "1 (TN) cal"=1.0, "2 (A) cal"=1.0, "2 (V) cal"=1.0, "2 (PF) cal"=1.0, "2 (TL) cal"=1.0, "2 (TN) cal"=1.0} ("CAL LAB01") -> [_ _ w3856 w3884 w3912 w3940 w3968 _]
                  tunnel: w3727 -> [_ _ _ _ _ _ _ w3974]
                  tunnel: w3726 -> [w3783 _ _ _ _ _ _ _]
                  tunnel: w3724 -> [_ w3810 _ _ _ _ _ _]
                  frame #0 {
                    n2154 = Index Array(array=w3783, index=2) -> (element=w3778:bool)
                    n2155 = Index Array(array=w3783, index=1) -> (element=w3779:bool)
                    n2156 = Index Array(array=w3783, index=0) -> (element=w3780:bool)
                    n2157 = local write "Error USB #2"(w3778) -> ()
                    n2158 = local write "Error USB #0"(w3780) -> ()
                    n2159 = local write "Error USB #1"(w3779) -> ()
                    n2160 = stacked-sequence {
                      tunnel: w3780 -> [w3787 _ _ _]
                      tunnel: w3779 -> [_ w3792 _ _]
                      tunnel: 0 -> [w3786 w3791 w3796 _]
                      tunnel: w3778 -> [_ _ w3797 _]
                      frame #0 {
                        n2161 = case shown="True" w3787 {
                          tunnel: w3786 -> [w3788 _]
                          frame False {
                            n2162 = local write "Er USB#0"(w3788) -> ()
                          }
                          frame True {
                            n2163 = local read "Er USB#0"() -> (w3790:dbl)
                            n2164 = Increment(x=w3790) -> (x+1=→"Er USB#0":dbl)
                          }
                        }
                      }
                      frame #1 {
                        n2165 = case shown="True" w3792 {
                          tunnel: w3791 -> [w3793 _]
                          frame False {
                            n2166 = local write "Er USB#1"(w3793) -> ()
                          }
                          frame True {
                            n2167 = local read "Er USB#1"() -> (w3795:dbl)
                            n2168 = Increment(x=w3795) -> (x+1=→"Er USB#1":dbl)
                          }
                        }
                      }
                      frame #2 {
                        n2169 = case shown="True" w3797 {
                          tunnel: w3796 -> [w3798 _]
                          frame False {
                            n2170 = local write "Er USB#2"(w3798) -> ()
                          }
                          frame True {
                            n2171 = local read "Er USB#2"() -> (w3800:dbl)
                            n2172 = Increment(x=w3800) -> (x+1=→"Er USB#2":dbl)
                          }
                        }
                      }
                      frame #3 {
                        w3806 = 10
                        n2173 = local read "Er USB#2"() -> (w3807:dbl)
                        n2174 = local read "Er USB#0"() -> (w3809:dbl)
                        n2175 = local read "Er USB#1"() -> (w3808:dbl)
                        n2176 = Greater Or Equal?(x=w3809, y=w3806) -> (x >= y?=w3804:bool)
                        n2177 = Greater Or Equal?(x=w3808, y=w3806) -> (x >= y?=w3803:bool)
                        n2178 = Greater Or Equal?(x=w3807, y=w3806) -> (x >= y?=w3802:bool)
                        n2179 = Or(x=w3804, y=w3803) -> (x .or. y?=w3805:bool)
                        n2180 = Or(x=w3805, y=w3802) -> (x .or. y?=→"Analog error":bool)
                      }
                    }
                  }
                  frame #1 {
                    # "display graph data on ADM page"
                    n2181 = local write "AI loop time"(w3810) -> ()
                    n2182 = local write "AI"(TRUE) -> ()
                    n2183 = Index Array(array=w3831, index=6) -> (element=→"LAB04-1 (GRAPH)":dynamicdata)
                    n2184 = Index Array(array=w3831, index=7) -> (element=→"LAB04-2 (GRAPH)":dynamicdata)
                    n2185 = Index Array(array=w3831, index=9) -> (element=→"LAB05-2 (GRAPH)":dynamicdata)
                    n2186 = Index Array(array=w3831, index=8) -> (element=→"LAB05-1 (GRAPH)":dynamicdata)
                    n2187 = Index Array(array=w3831, index=5) -> (element=→"LAB03-2 (GRAPH)":dynamicdata)
                    n2188 = Index Array(array=w3831, index=0) -> (element=→"LAB01-1 (GRAPH)":dynamicdata)
                    n2189 = Index Array(array=w3831, index=1) -> (element=→"LAB01-2 (GRAPH)":dynamicdata)
                    n2190 = Index Array(array=w3831, index=2) -> (element=→"LAB02-1 (GRAPH)":dynamicdata)
                    n2191 = Index Array(array=w3831, index=3) -> (element=→"LAB02-2 (GRAPH)":dynamicdata)
                    n2192 = Index Array(array=w3831, index=4) -> (element=→"LAB03-1 (GRAPH)":dynamicdata)
                  }
                  frame #2 {
                    n2193 = case shown="False" w3857 {
                      tunnel: [w3859 w3860] -> w3855
                      tunnel: w3856 -> [_ w3860]
                      frame False {
                        n2194 = local read "CAL LAB01"() -> (w3859:T15)
                      }
                      frame True {
                      }
                    }
                    n2195 = Unbundle By Name(w3858) -> ("OFF amps"=w3854:dbl, "VOLTS"=w3853:dbl, "PF"=w3852:dbl, "OFF amps"=w3851:dbl, "VOLTS"=w3850:dbl, "PF"=w3849:dbl)
                    n2196 = Unbundle By Name(w3855) -> ("1  (A) cal"=w3848:dbl, "1 (V) cal"=w3847:dbl, "1 (PF) cal"=w3846:dbl, "2 (A) cal"=w3845:dbl, "2 (V) cal"=w3844:dbl, "2 (PF) cal"=w3843:dbl)  [unwired: 4 out]
                    n2197 = Multiply(x=w3854, y=w3848) -> (x*y=w3841:dbl)
                    n2198 = Multiply(x=w3853, y=w3847) -> (x*y=w3840:dbl)
                    n2199 = Multiply(x=w3852, y=w3846) -> (x*y=w3839:dbl)
                    n2200 = Multiply(x=w3851, y=w3845) -> (x*y=w3837:dbl)
                    n2201 = Multiply(x=w3850, y=w3844) -> (x*y=w3836:dbl)
                    n2202 = Multiply(x=w3849, y=w3843) -> (x*y=w3835:dbl)
                    n2203 = local read "SIG LAB01-2"() -> (w3838:T2)
                    n2204 = local read "SIG LAB01-1"() -> (w3842:T2)
                    n2205 = Bundle By Name(cluster=w3842, "AMPS"=w3841, "VOLTS"=w3840, "PF"=w3839) -> (w3834:T2)
                    n2206 = Bundle By Name(cluster=w3838, "AMPS"=w3837, "VOLTS"=w3836, "PF"=w3835) -> (w3833:T2)
                    n2207 = global write "Global display 1.vi" "SIG LAB01-2"(w3833) -> ()
                    n2208 = global write "Global display 1.vi" "SIG LAB01-1"(w3834) -> ()
                    n2209 = local write "SIG LAB01-2"(w3833) -> ()
                    n2210 = local write "SIG LAB01-1"(w3834) -> ()
                  }
                  frame #3 {
                    n2211 = Unbundle By Name(w3886) -> ("OFF amps"=w3882:dbl, "VOLTS"=w3881:dbl, "PF"=w3880:dbl, "OFF amps"=w3879:dbl, "VOLTS"=w3878:dbl, "PF"=w3877:dbl)
                    n2212 = case shown="True" w3885 {
                      tunnel: [w3887 w3888] -> w3883
                      tunnel: w3884 -> [_ w3888]
                      frame False {
                        n2213 = local read "CAL LAB02"() -> (w3887:T16)
                      }
                      frame True {
                      }
                    }
                    n2214 = Unbundle By Name(w3883) -> ("1  (A) cal"=w3876:dbl, "1 (V) cal"=w3875:dbl, "1 (PF) cal"=w3874:dbl, "2 (A) cal"=w3873:dbl, "2 (V) cal"=w3872:dbl, "2 (PF) cal"=w3871:dbl)  [unwired: 4 out]
